vi "Get Just Validate.vi"(8 "error in (no error)":errorcluster, 11 "CFG JSON Base in":refnum<class "CFG JSON.lvclass">) -> (0 "error out":errorcluster, 2 "Just Validate":bool, 3 "CFG JSON Base out":refnum<class "CFG JSON.lvclass">)   [LabVIEW 2023, in "HAL GOOP4.lvlib" / "CFG JSON.lvclass"]
uses:
  CFG JSON.lvclass
  CFG JSON.lvclass/CFG JSON.ctl
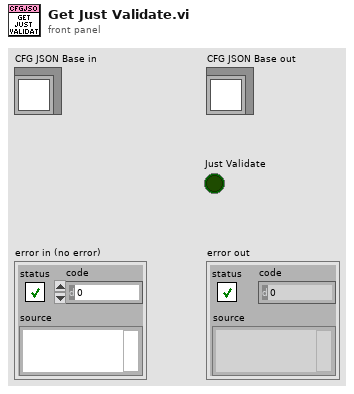
[diagram p1: front panel]
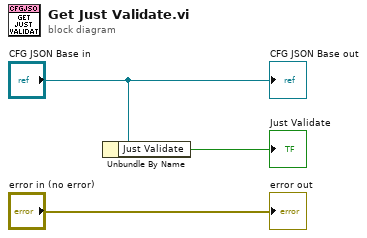
[diagram p0: block diagram]
diagram:
  n1 = Unbundle By Name("CFG JSON Base in") -> ("Just Validate"=→"Just Validate":bool)
  "error out" <- "error in (no error)"
  "CFG JSON Base out" <- "CFG JSON Base in"
